vi "Vpp to Amplitude and Offset.vi"(5 "Vpp":dbl) -> (0 "Amplitude":dbl, 1 "Offset":dbl)   [LabVIEW 2014]
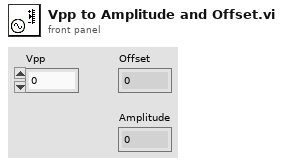
[diagram p1: front panel]
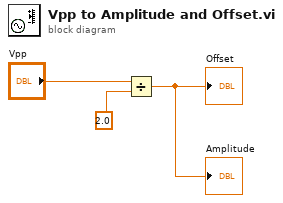
[diagram p0: block diagram]
diagram:
  n1 = Divide(x="Vpp", y=2.0) -> (x/y=→"Offset" →"Amplitude":dbl)
